vi "TIn.VI"(2 "Options (FILTER)":bool=TRUE, 3 "Scale":u32(ring) items=["CELSIUS", "FAHRENHEIT", "KELVIN"], 4 "Chan":u32, 5 "BoardNum (0)":u32 max=8) -> (0 "ErrCode":i32, 1 "Temperature":sgl format="%.2f")   [LabVIEW 2019, in "DAQ_Engine.lvclass"]
doc: "Developed by Kevin Thompson\nkevin@thompsonengineering.net\n\nCopyright 2020\nThompson Engineering, LLC\nReads an analog input channel, linearizes it according to the sensor type, and returns the temperature in degrees."
uses:
  DAQ_Engine.lvclass
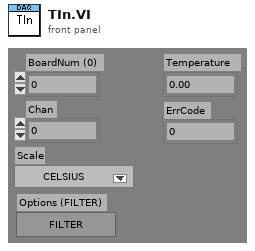
[diagram p1: front panel]
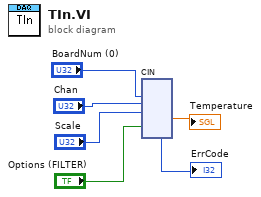
[diagram p0: block diagram]
diagram:
  n1 = cin("BoardNum (0)", "Chan", "Scale", "Options (FILTER)") -> (→"Temperature":sgl, →"ErrCode":i32)  [unwired: 6 in]
